vi "Execute.vi"(5 "Init user event out":refnum<user-event>, 7 "user event in":refnum<user-event>, 8 "Advanced Waveform In":refnum<class "Advanced Waveform.lvclass">, 9 "Initialise in":refnum<class "Initialise.lvclass">, 10 "Command Queue":refnum<queue>, 11 "error in (no error)":errorcluster) -> (0 "Advanced Waveform Out":refnum<class "Advanced Waveform.lvclass">, 1 "Initialise out":refnum<class "Initialise.lvclass">, 2 "Stop":bool, 3 "error out":errorcluster)   [LabVIEW 2011, in "Initialise.lvclass"]
uses:
  Initialise.lvclass
  Advanced Waveform Class/Advanced Waveform.lvclass
  Message.lvclass
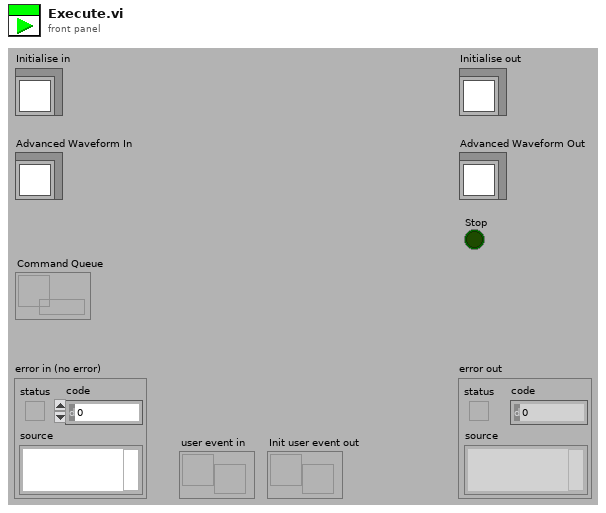
[diagram p1: front panel]
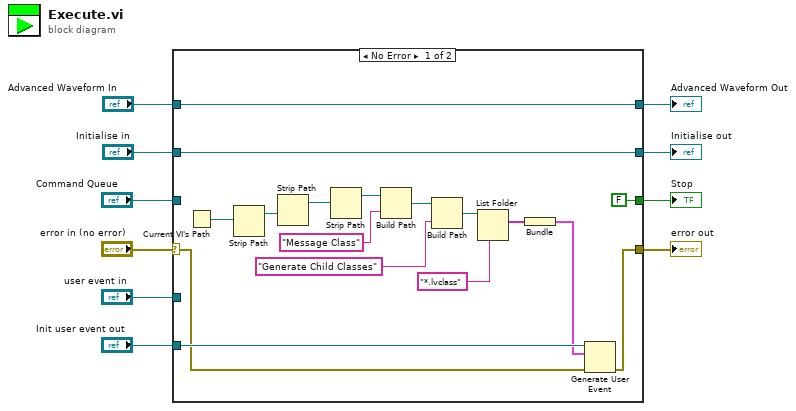
[diagram p0: block diagram]
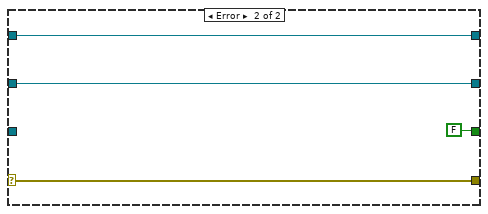
[diagram p2: hidden frame]
diagram:
  n1 = case shown="No Error" "error in (no error)" {
    selector: "error in (no error)" -> [w23 w29]
    tunnel: "Command Queue" -> [_ _]
    tunnel: [w26 w31] -> w8
    tunnel: "Initialise in" -> [w26 w31]
    tunnel: [w27 w30] -> w6
    tunnel: "Advanced Waveform In" -> [w27 w30]
    tunnel: "user event in" -> [_ _]
    tunnel: "Init user event out" -> [w24 _]
    tunnel: [w22 w29] -> w2
    tunnel: [FALSE FALSE] -> w1
    frame No Error {
      n2 = Current VI's Path() -> (path=w21:path)
      n3 = Strip Path(path=w21) -> (stripped path=w20:path)  [unwired: 1 out]
      n4 = Strip Path(path=w20) -> (stripped path=w19:path)  [unwired: 1 out]
      n5 = Strip Path(path=w19) -> (stripped path=w17:path)  [unwired: 1 out]
      n6 = Build Path(base path=w17, name or relative path="Message Class") -> (appended path=w15:path)
      n7 = Build Path(base path=w15, name or relative path="Generate Child Classes") -> (appended path=w13:path)
      n8 = List Folder(path=w13, pattern="*.lvclass") -> (filenames=w11:string[])  [unwired: 2 in, 3 out]
      n9 = Bundle("filenames"=w11) -> (w18:cluster{"filenames":string[]})  [unwired: 1 in]
      n10 = Generate User Event(user event=w24, event data cluster=w18, error in=w23) -> (error out=w22:errorcluster)  [unwired: 1 out]
    }
    frame Error {
    }
  }
  "error out" <- w2
  "Initialise out" <- w8
  "Stop" <- w1
  "Advanced Waveform Out" <- w6
